vi "RSZVB Set Simultaneous Measurement Minimum Frequency Offset Direct.vi"(8 "error in (no error)":errorcluster {"code" format="%.0x"}, 9 "Minimum Frequency Offset (1)":i32=1, 10 "Channel (1)":i32=1, 11 "VISA resource name":refnum<visa-resource-name>) -> (0 "error out":errorcluster {"code" format="%.0x"}, 3 "VISA resource name out":refnum<visa-resource-name>)   [LabVIEW 2011]
doc: "This VI directly specifies the minimum frequency offset in DIRect mode.\n\nRemote-control command(s):\nSOURce<Ch>:GROup:SIMultaneous:FOFFset:MOFFset:DVALue"
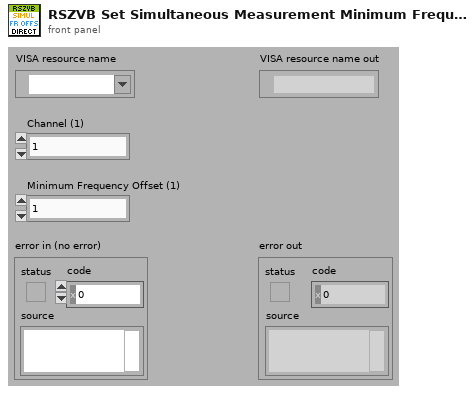
[diagram p1: front panel]
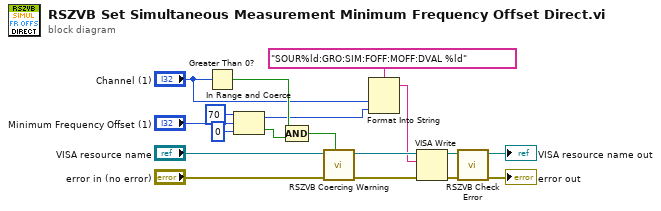
[diagram p0: block diagram]
diagram:
  n1 = Greater Than 0?(x="Channel (1)") -> (x > 0?=w8:bool)
  n2 = In Range and Coerce(upper limit=70, x="Minimum Frequency Offset (1)", lower limit=0) -> (coerced(x)=w7:i32, In Range?=w13:bool)
  n3 = Compound Arithmetic op=AND(w8, w13) -> (w12:bool)
  n4 = call "RSZVB Coercing Warning.vi"("In Range?"=w12, "error in (no error)"="error in (no error)", "VISA session"="VISA resource name") -> ("error out"=w16:errorcluster, "dup VISA session"=w17:refnum<visa-resource-name>)  [unwired: 7 in]
  n5 = Format Into String(format string="SOUR%ld:GRO:SIM:FOFF:MOFF:DVAL %ld", "Channel (1)", w7) -> (resulting string=w11:string)  [unwired: 2 in, 1 out]
  n6 = VISA Write(VISA resource name=w17, write buffer=w11, error in (no error)=w16) -> (VISA resource name out=w14:refnum<visa-resource-name>, error out=w15:errorcluster)  [unwired: 1 out]
  n7 = call "RSZVB Check Error.vi"("error in (no error)"=w15, "VISA session"=w14) -> ("error out"=→"error out":errorcluster, "dup VISA session"=→"VISA resource name out":refnum<visa-resource-name>)  [unwired: 8 in]
